vi "TwGetRegUserDataFromH5LV.vi"(0 "filename":string, 1 "location":string, 2 "bufIndex":i32, 3 "writeIndex":i32, 4 "error in (no error)":errorcluster) -> (5 "error out":errorcluster, 6 "buffer out":dbl[](array[numeric]), 7 "Array":string[](array[string]))   [LabVIEW 2009]
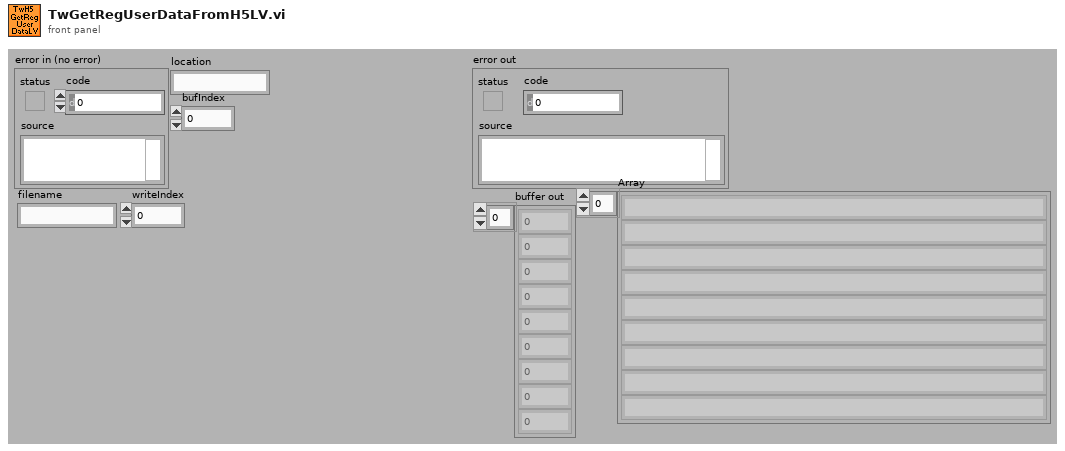
[diagram p1: front panel]
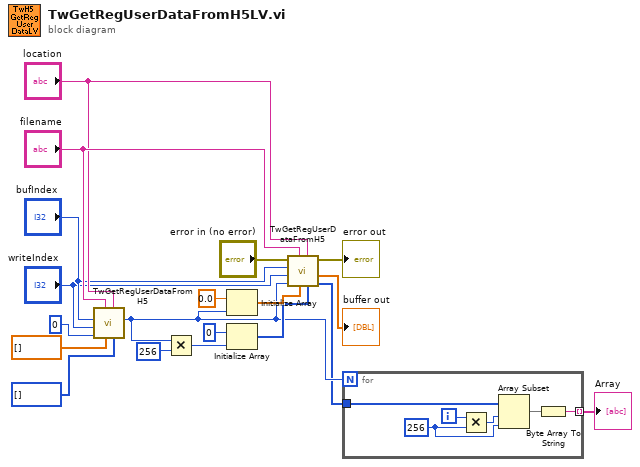
[diagram p0: block diagram]
diagram:
  n1 = call "TwGetRegUserDataFromH5.vi"("description in"=u8[] [], "location"="location", "buffer in"=dbl[] [], "filename"="filename", "bufLength in"=0, "writeIndex"="writeIndex", "bufIndex"="bufIndex") -> ("bufLength out"=w4:i32)  [unwired: 1 in, 3 out]
  n2 = Multiply(x=w4, y=256) -> (x*y=w5:i32)
  n3 = Initialize Array(0.0 ("element"), w4) -> (w10:dbl[])
  n4 = Initialize Array(u8 0 ("element"), w5) -> (w7:u8[])
  n5 = call "TwGetRegUserDataFromH5.vi"("description in"=w7, "location"="location", "buffer in"=w10, "filename"="filename", "bufLength in"=w4, "writeIndex"="writeIndex", "bufIndex"="bufIndex", "error in (no error)"="error in (no error)") -> ("description out"=w3:u8[], "buffer out"=→"buffer out":dbl[], "error out"=→"error out":errorcluster)  [unwired: 1 out]
  n6 = for {
    N: w4 -> [_]
    tunnel: w3 -> [w25]
    tunnel: [w21] -> w2 mode=indexing
    i -> [w24]
    w23 = 256 ("length")
    n7 = Multiply(x=w24, y=w23) -> (x*y=w22:i32)
    n8 = Array Subset(array=w25, index=w22, length=w23) -> (w20:u8[])
    n9 = Byte Array To String(unsigned byte array=w20) -> (string=w21:string)
  }
  "Array" <- w2
